vi "Get Baseline Image.vi"() -> (3 "Image Out":T1)   [LabVIEW 2011]
uses:
  <vilib>/vision/Image Controls.llb/IMAQ Image.ctl
panel:
  out "File Exists?":bool
  out "error out":errorcluster
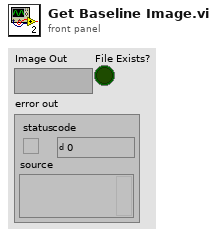
[diagram p1: front panel]
types:
  T1 = typedef "IMAQ Image.ctl" = refnum<image>
  T2 = typedef "Image Type" = u32
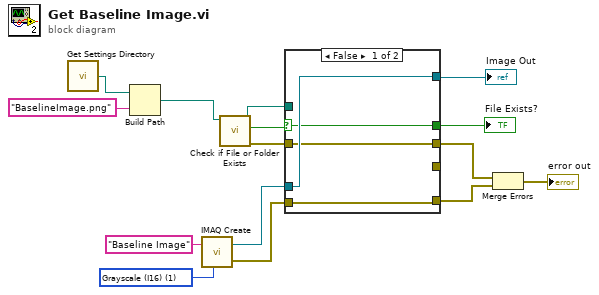
[diagram p0: block diagram]
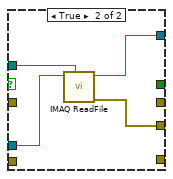
[diagram p2: hidden frame]
diagram:
  w13 = T2 1 items=["Grayscale (U8)", "Grayscale (I16)", "Grayscale (SGL)", "Complex (CSG)", "RGB (U32)", "HSL (U32)", "RGB (U64)", "Grayscale (U16)"] ("Image Type")
  n1 = call "Get Settings Directory.vi"() -> ("Settings Folder Path"=w2:path)  [unwired: 5 in]
  n2 = Build Path(base path=w2, name or relative path="BaselineImage.png") -> (appended path=w1:path)
  n3 = call "IMAQ Create"("Image Name"="Baseline Image", "Image Type"=w13) -> ("New Image"=w15:T1, "error out"=w9:errorcluster)  [unwired: 3 in]
  n4 = call <vilib>:"Check if File or Folder Exists.vi"("path"=w1) -> ("error out"=w8:errorcluster, "file or folder exists?"=w11:bool, "dup path"=w10:path)  [unwired: 8 in]
  n5 = case shown="False" w11 {
    selector: w11 -> [w16 _]
    tunnel: w15 -> [w19 w23]
    tunnel: [w19 w22] -> w12
    tunnel: [_ w21] -> _
    tunnel: w10 -> [_ w20]
    tunnel: w9 -> [w17 _]
    tunnel: w8 -> [w18 _]
    tunnel: [w18 _] -> w7
    tunnel: [w17 _] -> w6
    tunnel: [w16 _] -> w4
    frame False {
    }
    frame True {
      n6 = call "IMAQ ReadFile"("File Path"=w20, "Image"=w23) -> ("error out"=w21:errorcluster, "Image Out"=w22:T1)  [unwired: 5 in, 3 out]
    }
  }
  "Image Out" <- w12
  "File Exists?" <- w4
  n7 = Merge Errors(w7, w6) -> (→"error out":errorcluster)
